vi "ScanSteuerung_sort.vi"(1 "ScanSteuerung":T1=[{"Time [s]"=0.0, "action"=enum."Abs", "channel"=enum."SMoveTime", "value (/s)"=0.00096}, {"Time [s]"=0.0, "action"=enum."Abs", "channel"=enum."GalvoX", "value (/s)"=-0.0005171784141124036}, {"Time [s]"=0.0, "action"=enum."Abs", "channel"=enum."GalvoY", "value (/s)"=-0.0005424121424136167}, {"Time [s]"=0.0, "action"=enum."Abs", "channel"=enum."Galvo3", "value (/s)"=0.0}, {"Time [s]"=0.0, "action"=enum."Abs", "channel"=enum."Image1X", "value (/s)"=0.0}, {"Time [s]"=0.0, "action"=enum."Abs", "channel"=enum."Image1Y", "value (/s)"=0.0}, {"Time [s]"=0.0, "action"=enum."Abs", "channel"=enum."Digital", "value (/s)"=2.0}, {"Time [s]"=0.0, "action"=enum."LoopStart", "channel"=enum."Loop", "value (/s)"=250.0}, {"Time [s]"=0.0, "action"=enum."Inc", "channel"=enum."GalvoX", "value (/s)"=0.0833334166669957}, {"Time [s]"=0.0, "action"=enum."Inc", "channel"=enum."GalvoY", "value (/s)"=0.0}, {"Time [s]"=0.0, "action"=enum."Inc", "channel"=enum."Galvo3", "value (/s)"=41666.666666666664}, {"Time [s]"=2.4e-05, "action"=enum."Inc", "channel"=enum."Image1X", "value (/s)"=41666.666666666664}, {"Time [s]"=0.012, "action"=enum."Abs", "channel"=enum."Digital", "value (/s)"=3.0}, {"Time [s]"=0.012, "action"=enum."Inc", "channel"=enum."GalvoX", "value (/s)"=0.0}, {"Time [s]"=0.012, "action"=enum."Inc", "channel"=enum."GalvoY", "value (/s)"=0.04166670833349785}, {"Time [s]"=0.012, "action"=enum."Inc", "channel"=enum."Galvo3", "value (/s)"=0.0}, {"Time [s]"=0.012, "action"=enum."Inc", "channel"=enum."Image1X", "value (/s)"=0.0}, {"Time [s]"=0.012048, "action"=enum."Abs", "channel"=enum."Digital", "value (/s)"=2.0}, {"Time [s]"=0.012048, "action"=enum."Rel", "channel"=enum."Image1Y", "value (/s)"=1.0}, {"Time [s]"=0.012048, "action"=enum."Inc", "channel"=enum."GalvoX", "value (/s)"=-0.0833334166669957}, {"Time [s]"=0.012048, "action"=enum."Inc", "channel"=enum."GalvoY", "value (/s)"=-0.0}, {"Time [s]"=0.012048, "action"=enum."Inc", "channel"=enum."Galvo3", "value (/s)"=-41666.666666666664}, {"Time [s]"=0.012072, "action"=enum."Inc", "channel"=enum."Image1X", "value (/s)"=-41666.666666666664}, {"Time [s]"=0.024048, "action"=enum."Abs", "channel"=enum."Digital", "value (/s)"=3.0}, {"Time [s]"=0.024048, "action"=enum."Inc", "channel"=enum."GalvoX", "value (/s)"=0.0}, {"Time [s]"=0.024048, "action"=enum."Inc", "channel"=enum."GalvoY", "value (/s)"=0.04166670833349785}, {"Time [s]"=0.024048, "action"=enum."Inc", "channel"=enum."Galvo3", "value (/s)"=0.0}, {"Time [s]"=0.024048, "action"=enum."Inc", "channel"=enum."Image1X", "value (/s)"=0.0}, {"Time [s]"=0.024096, "action"=enum."Abs", "channel"=enum."Digital", "value (/s)"=2.0}, {"Time [s]"=0.024096, "action"=enum."Rel", "channel"=enum."Image1Y", "value (/s)"=1.0}, {"Time [s]"=0.024096, "action"=enum."LoopEnd", "channel"=enum."Loop", "value (/s)"=0.0}, {"Time [s]"=6.024, "action"=enum."Inc", "channel"=enum."GalvoX", "value (/s)"=0.0}, {"Time [s]"=6.024, "action"=enum."Inc", "channel"=enum."GalvoY", "value (/s)"=0.0}, {"Time [s]"=6.024, "action"=enum."Inc", "channel"=enum."Galvo3", "value (/s)"=0.0}, {"Time [s]"=6.024, "action"=enum."Abs", "channel"=enum."Digital", "value (/s)"=0.0}]) -> (0 "ScanSteuerung":T1=[{"Time [s]"=0.0, "action"=enum."Abs", "channel"=enum."SMoveTime", "value (/s)"=0.00096}, {"Time [s]"=0.0, "action"=enum."Abs", "channel"=enum."GalvoX", "value (/s)"=-0.0005171784141124036}, {"Time [s]"=0.0, "action"=enum."Abs", "channel"=enum."GalvoY", "value (/s)"=-0.0005424121424136167}, {"Time [s]"=0.0, "action"=enum."Abs", "channel"=enum."Galvo3", "value (/s)"=0.0}, {"Time [s]"=0.0, "action"=enum."Abs", "channel"=enum."Image1X", "value (/s)"=0.0}, {"Time [s]"=0.0, "action"=enum."Abs", "channel"=enum."Image1Y", "value (/s)"=0.0}, {"Time [s]"=0.0, "action"=enum."Abs", "channel"=enum."Digital", "value (/s)"=2.0}, {"Time [s]"=0.0, "action"=enum."LoopStart", "channel"=enum."Loop", "value (/s)"=250.0}, {"Time [s]"=0.0, "action"=enum."Inc", "channel"=enum."GalvoX", "value (/s)"=0.0833334166669957}, {"Time [s]"=0.0, "action"=enum."Inc", "channel"=enum."GalvoY", "value (/s)"=0.0}, {"Time [s]"=0.0, "action"=enum."Inc", "channel"=enum."Galvo3", "value (/s)"=41666.666666666664}, {"Time [s]"=2.4e-05, "action"=enum."Inc", "channel"=enum."Image1X", "value (/s)"=41666.666666666664}, {"Time [s]"=0.012, "action"=enum."Abs", "channel"=enum."Digital", "value (/s)"=3.0}, {"Time [s]"=0.012, "action"=enum."Inc", "channel"=enum."GalvoX", "value (/s)"=0.0}, {"Time [s]"=0.012, "action"=enum."Inc", "channel"=enum."GalvoY", "value (/s)"=0.04166670833349785}, {"Time [s]"=0.012, "action"=enum."Inc", "channel"=enum."Galvo3", "value (/s)"=0.0}, {"Time [s]"=0.012, "action"=enum."Inc", "channel"=enum."Image1X", "value (/s)"=0.0}, {"Time [s]"=0.012048, "action"=enum."Abs", "channel"=enum."Digital", "value (/s)"=2.0}, {"Time [s]"=0.012048, "action"=enum."Rel", "channel"=enum."Image1Y", "value (/s)"=1.0}, {"Time [s]"=0.012048, "action"=enum."Inc", "channel"=enum."GalvoX", "value (/s)"=-0.0833334166669957}, {"Time [s]"=0.012048, "action"=enum."Inc", "channel"=enum."GalvoY", "value (/s)"=-0.0}, {"Time [s]"=0.012048, "action"=enum."Inc", "channel"=enum."Galvo3", "value (/s)"=-41666.666666666664}, {"Time [s]"=0.012072, "action"=enum."Inc", "channel"=enum."Image1X", "value (/s)"=-41666.666666666664}, {"Time [s]"=0.024048, "action"=enum."Abs", "channel"=enum."Digital", "value (/s)"=3.0}, {"Time [s]"=0.024048, "action"=enum."Inc", "channel"=enum."GalvoX", "value (/s)"=0.0}, {"Time [s]"=0.024048, "action"=enum."Inc", "channel"=enum."GalvoY", "value (/s)"=0.04166670833349785}, {"Time [s]"=0.024048, "action"=enum."Inc", "channel"=enum."Galvo3", "value (/s)"=0.0}, {"Time [s]"=0.024048, "action"=enum."Inc", "channel"=enum."Image1X", "value (/s)"=0.0}, {"Time [s]"=0.024096, "action"=enum."Abs", "channel"=enum."Digital", "value (/s)"=2.0}, {"Time [s]"=0.024096, "action"=enum."Rel", "channel"=enum."Image1Y", "value (/s)"=1.0}, {"Time [s]"=0.024096, "action"=enum."LoopEnd", "channel"=enum."Loop", "value (/s)"=0.0}, {"Time [s]"=6.024, "action"=enum."Inc", "channel"=enum."GalvoX", "value (/s)"=0.0}, {"Time [s]"=6.024, "action"=enum."Inc", "channel"=enum."GalvoY", "value (/s)"=0.0}, {"Time [s]"=6.024, "action"=enum."Inc", "channel"=enum."Galvo3", "value (/s)"=0.0}, {"Time [s]"=6.024, "action"=enum."Abs", "channel"=enum."Digital", "value (/s)"=0.0}])   [LabVIEW 2011]
uses:
  ScanControl.ctl
  ScanControl_Action.ctl
  ScanControl_Channel.ctl
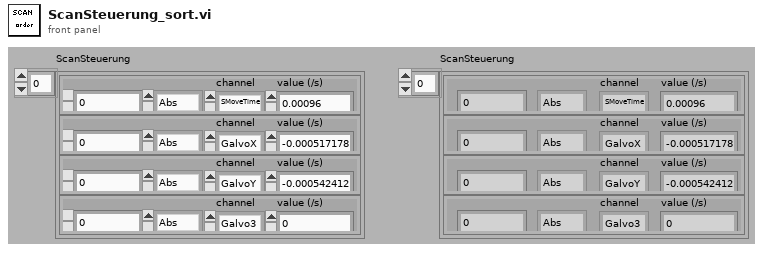
[diagram p1: front panel]
types:
  T1 = typedef "ScanControl.ctl" = cluster{"Time [s]":dbl, "action":T2, "channel":T3, "value (/s)":dbl}[]
  T2 = typedef "ScanControl_Action.ctl" = enum16{"Abs", "Rel", "Inc", "IncInc", "LoopStart", "LoopEnd", "WaitTriggerRising"}
  T3 = typedef "ScanControl_Channel.ctl" = enum16{"Com", "AnalogConfig", "AnalogValue", "GalvoX", "GalvoY", "Galvo3", "Galvo4", "Digital", "Free", "Loop", "SMoveTime", "Image1X", "Image1Y", "Image2X", "Image2Y"}
  T4 = cluster{"Time [s]":dbl, "action":T2, "channel":T3, "value (/s)":dbl}
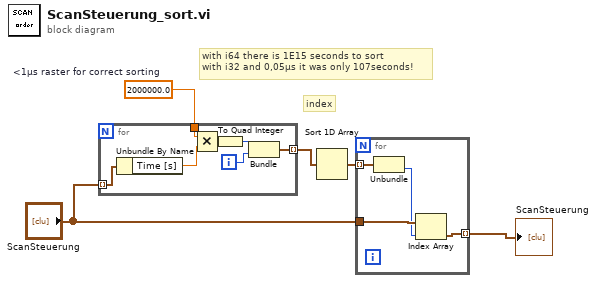
[diagram p0: block diagram]
diagram:
  w4 = 2000000.0  # <1µs raster for correct sorting
  # "with i64 there is 1E15 seconds to sort\nwith i32 and 0,05µs it was only 107seconds!"
  # "index"
  n1 = for {
    tunnel: "ScanSteuerung" -> [w12] mode=indexing
    tunnel: w4 -> [w11]
    tunnel: [w7] -> w2 mode=indexing
    i -> [w8]
    n2 = Unbundle By Name(w12) -> ("Time [s]"=w10:dbl)
    n3 = Multiply(x=w11, y=w10) -> (x*y=w6:dbl)
    n4 = To Quad Integer(1:w6) -> (0:w9:i64)
    n5 = Bundle(w9, w8) -> (w7:cluster{i64, i32})  [unwired: 1 out]
  }
  n6 = Sort 1D Array(array=w2) -> (sorted array=w5:cluster{i64, i32}[])
  n7 = for {
    tunnel: w5 -> [w14] mode=indexing
    tunnel: [w16] -> w1 mode=indexing
    tunnel: "ScanSteuerung" -> [w15]
    n8 = Unbundle(w14) -> (w13:i32)  [unwired: 1 out]
    n9 = Index Array(array=w15, index=w13) -> (element=w16:T4)
  }
  "ScanSteuerung" <- w1
